vi "3-Buttons HamburgerVI.vi"(8 "error in (no error)":errorcluster, 9 "Context":variant, 10 "HamburgerItemClicked Event":refnum<user-event>, 11 "HamburgerCtl Ref":refnum<vi>) -> ()   [LabVIEW 2017]
uses:
  Hamburger Menu Library.lvlib
panel:
  in  "Item1":bool
  in  "Item2":bool
  in  "Item3":bool
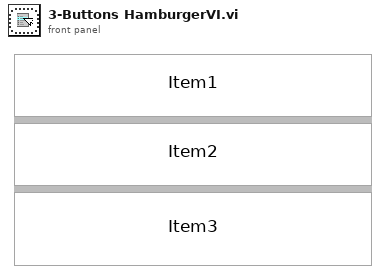
[diagram p1: front panel]
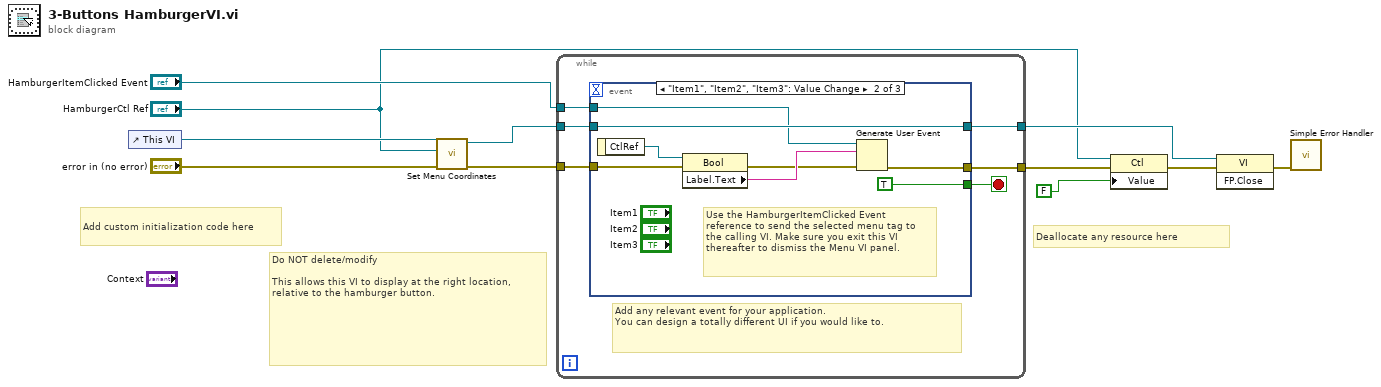
[diagram p0: block diagram]
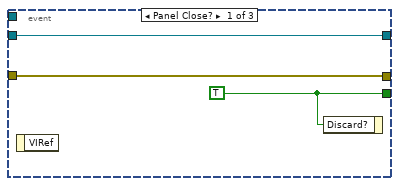
[diagram p2: hidden frame]
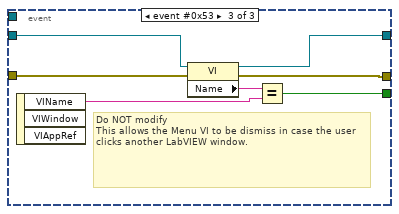
[diagram p3: hidden frame]
diagram:
  # "Deallocate any resource here"
  # "Add custom initialization code here"
  # "Do NOT delete/modify\n\nThis allows this VI to display at the right location, relative to the hamburger button."
  n1 = control-ref of="This VI"() -> (w11:refnum<vi>)
  n2 = call "Set Menu Coordinates.vi"("error in (no error)"="error in (no error)", "HamburgerCtl Ref"="HamburgerCtl Ref", "VI in"=w11) -> ("error out"=w9:errorcluster, "VI out"=w8:refnum<vi>)  [unwired: 7 in]
  n3 = while {
    tunnel: [w14] -> w10
    tunnel: w8 -> [w16]
    tunnel: w9 -> [w15]
    tunnel: [w13] -> w3
    tunnel: "HamburgerItemClicked Event" -> [w12]
    stop <- w17 stop-if-true
    # "Add any relevant event for your application.\nYou can design a totally different UI if you would like to."
    n4 = event shown="[1] \"Item1\", \"Item2\", \"Item3\": Value Change" {
      selector: _ -> [_ _ _]
      dyn-events: _ -> [_ _ _]
      timeout: _ -> [_ _ _]
      tunnel: [w20 TRUE w34] -> w17
      tunnel: w16 -> [w19 w27 w33]
      tunnel: w15 -> [w18 w23 w31]
      tunnel: [w19 w27 w30] -> w14
      tunnel: [w18 w21 w29] -> w13
      tunnel: w12 -> [_ w26 _]
      event Panel Close? {
        w20 = TRUE ("Discard?")
        n5 = event-data() -> ()  [unwired: 1 in, 1 out]
        n6 = event-data("Discard?"=w20) -> ()  [unwired: 1 in, 1 out]
      }
      event "Item1", "Item2", "Item3": Value Change {
        # "Use the HamburgerItemClicked Event reference to send the selected menu tag to the calling VI. Make sure you exit this VI thereafter to dismiss the Menu VI panel."
        n7 = event-data() -> ("CtlRef"=w25:refnum<vi>)  [unwired: 1 in]
        n8 = property class="Bool"(reference=w25, error in=w23) -> (error out=w22:errorcluster, "Label.Text"=w24:string)  [unwired: 1 out]
        n9 = Generate User Event(user event=w26, event data cluster=w24, error in=w22) -> (error out=w21:errorcluster)  [unwired: 1 in, 1 out]
      }
      event event #0x53 {
        # "Do NOT modify\nThis allows the Menu VI to be dismiss in case the user clicks another LabVIEW window."
        n10 = event-data() -> ("VIName"=w35:string)  [unwired: 1 in, 2 out]
        n11 = property class="VI"(reference=w33, error in=w31) -> (reference out=w30:refnum<vi>, error out=w29:errorcluster, "Name"=w32:string)
        n12 = Equal?(x=w32, y=w35) -> (x = y?=w34:bool)
      }
    }
  }
  n13 = property class="Ctl"(reference="HamburgerCtl Ref", error in=w3, "Value"=FALSE) -> (error out=w2:errorcluster)  [unwired: 1 out]
  n14 = invoke class="VI" method="FP.Close"(reference=w10, error in=w2) -> (error out=w5:errorcluster)  [unwired: 1 in, 2 out]
  n15 = call <vilib>:"Simple Error Handler.vi"("error in (no error)"=w5) -> ()  [unwired: 4 in, 5 out]
